vi "GraphSetting Get ScaleName (XY).vi"(8 "error in (no error)":errorcluster caption="エラー入力（エラーなし）", 11 "XYグラフref(in)":refnum<vi>) -> (0 "error out":errorcluster caption="エラー出力", 1 "Y軸名称[]":string[](array[string]), 2 "X軸名称[]":string[](array[string]))   [LabVIEW 2016]
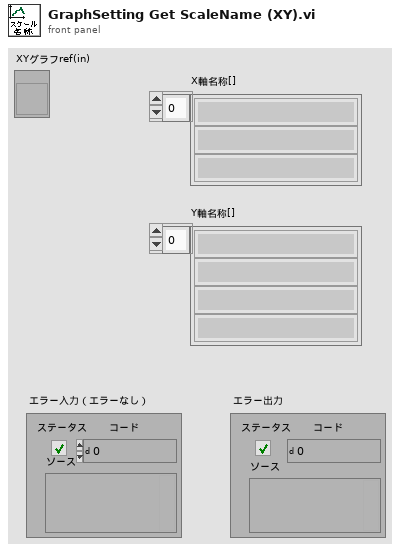
[diagram p1: front panel]
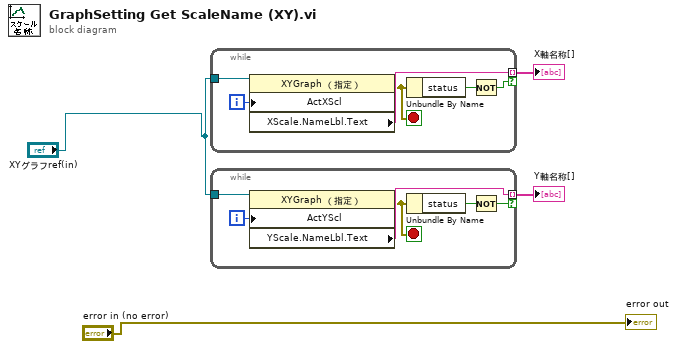
[diagram p0: block diagram]
diagram:
  n1 = while {
    tunnel: "XYグラフref(in)" -> [w10]
    tunnel: [w8] -> w4 mode=indexing if=w5
    i -> [w9]
    stop <- w7 stop-if-true
    n2 = property class="XYGraph （指定）"(reference=w10, "ActXScl"=w9) -> (error out=w7:errorcluster, "XScale.NameLbl.Text"=w8:string)  [unwired: 1 in, 1 out]
    n3 = Unbundle By Name(w7) -> ("status"=w6:bool)
    n4 = Not(x=w6) -> (.not. x?=w5:bool)
  }
  "X軸名称[]" <- w4
  n5 = while {
    tunnel: "XYグラフref(in)" -> [w16]
    tunnel: [w14] -> w3 mode=indexing if=w13
    i -> [w15]
    stop <- w12 stop-if-true
    n6 = property class="XYGraph （指定）"(reference=w16, "ActYScl"=w15) -> (error out=w12:errorcluster, "YScale.NameLbl.Text"=w14:string)  [unwired: 1 in, 1 out]
    n7 = Unbundle By Name(w12) -> ("status"=w11:bool)
    n8 = Not(x=w11) -> (.not. x?=w13:bool)
  }
  "Y軸名称[]" <- w3
  "error out" <- "error in (no error)"
